vi "flow data sim.vi"(1 "Boondoggle Input":dbl) -> (0 "Flowrate Data":T1(array[cluster]))   [LabVIEW 2018]
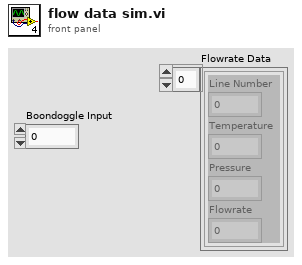
[diagram p1: front panel]
types:
  T1 = cluster{"Line Number":dbl, "Temperature":dbl, "Pressure":dbl, "Flowrate":dbl}[]
  T2 = cluster{"Line Number":dbl, "Temperature":dbl, "Pressure":dbl, "Flowrate":dbl}
  T3 = cluster{"[0]":dbl, "[1]":dbl, "[2]":dbl, "[3]":dbl}
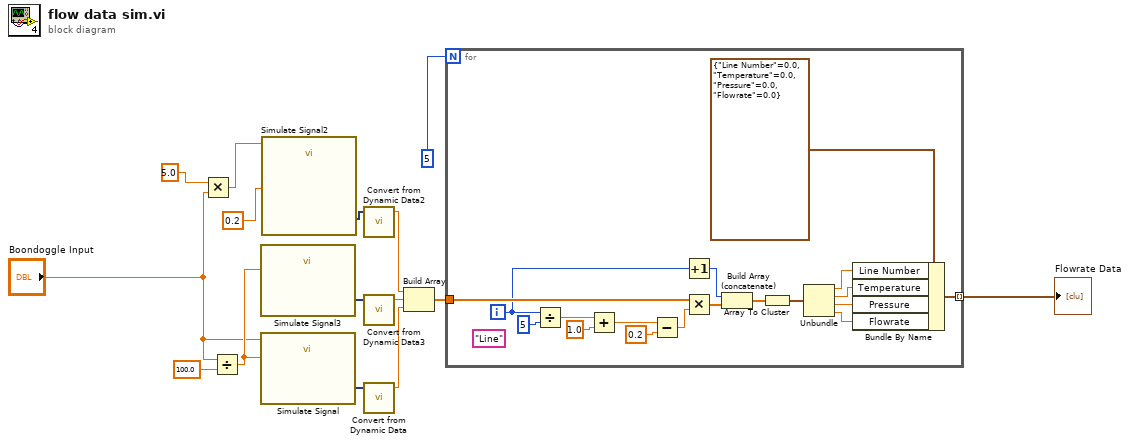
[diagram p0: block diagram]
diagram:
  n1 = Multiply(x=5.0 ("Offset"), y="Boondoggle Input") -> (x*y=w1:dbl)
  n2 = Divide(x="Boondoggle Input", y=100.0) -> (x/y=w4:dbl)
  n3 = call "Simulate Signal3"("Spectral amplitude"=w4) -> ("DC Pressure Signal"=w13:dynamicdata)  [unwired: 13 in, 1 out]
  n4 = call "Simulate Signal"("Offset"="Boondoggle Input", "Spectral amplitude"=w4) -> ("DC Flowrate Signal"=w11:dynamicdata)  [unwired: 12 in, 1 out]
  n5 = call "Simulate Signal2"("Offset"=w1, "Spectral amplitude"=0.2) -> ("DC Temperature Signal"=w12:dynamicdata)  [unwired: 12 in, 1 out]
  n6 = call "Convert from Dynamic Data2"("Dynamic Data Type"=w12) -> ("Scalar"=w10:dbl)  [unwired: 3 in]
  n7 = call "Convert from Dynamic Data3"("Dynamic Data Type"=w13) -> ("Scalar"=w9:dbl)  [unwired: 3 in]
  n8 = call "Convert from Dynamic Data"("Dynamic Data Type"=w11) -> ("Scalar"=w8:dbl)  [unwired: 3 in]
  n9 = Build Array(w10, w9, w8) -> (w6:dbl[])
  n10 = for {
    N: 5 -> [_]
    tunnel: w6 -> [w33]
    tunnel: [w19] -> w15 mode=indexing
    i -> [w17]
    (unwired) "Line"
    n11 = Divide(x=w17, y=5) -> (x/y=w31:dbl)
    n12 = Add(x=w31, y=1.0) -> (x+y=w29:dbl)
    n13 = Subtract(x=w29, y=0.2) -> (x-y=w27:dbl)
    n14 = Increment(x=w17) -> (x+1=w16:i32)
    n15 = Multiply(x=w33, y=w27) -> (x*y=w26:dbl[])
    n16 = Build Array (concatenate)(w16, w26) -> (w25:dbl[])
    n17 = Array To Cluster(array=w25) -> (cluster=w24:T3)
    n18 = Unbundle(w24) -> ("[0]"=w23:dbl, "[1]"=w22:dbl, "[2]"=w21:dbl, "[3]"=w20:dbl)
    n19 = Bundle By Name(cluster=T2 {"Line Number"=0.0, "Temperature"=0.0, "Pressure"=0.0, "Flowrate"=0.0}, "Line Number"=w23, "Temperature"=w22, "Pressure"=w21, "Flowrate"=w20) -> (w19:T2)
  }
  "Flowrate Data" <- w15
